vi "MW_AHRS_Paser.vi"(4 "error":errorcluster, 7 "String In":string) -> (0 "error IO":errorcluster, 3 "Output":T1)   [LabVIEW 2015]
panel:
  out "Yaw":dbl
  out "Pitch":dbl
  out "Roll":dbl
  out "Gyro_Z":dbl
  out "Gyro_Y":dbl
  out "Gyro_X":dbl
  out "Acc_X":dbl
  out "Acc_Y":dbl
  out "Acc_Z":dbl
  out "String":string
  # "MW-AHRS 프로그램 이며 센서 출력을 ACC, Gryo, 오일러 출력으로 \n세팅해야 프로그램이 정상적으로 구동 됨"
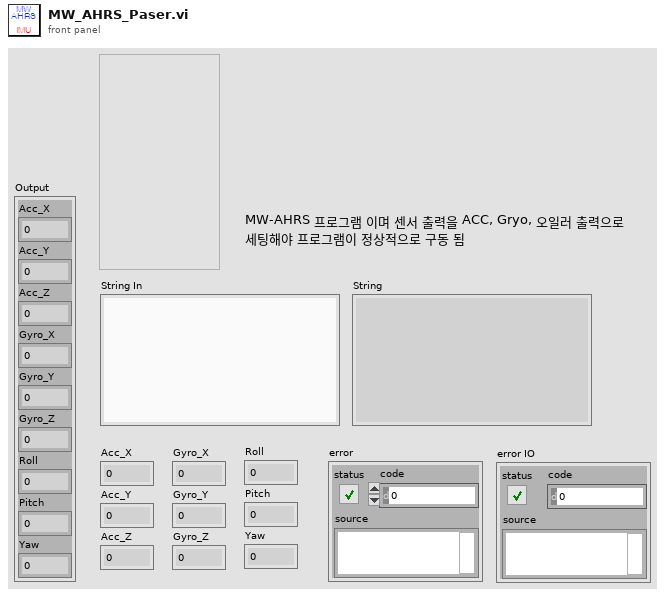
[diagram p1: front panel]
types:
  T1 = cluster{"Acc_X":dbl, "Acc_Y":dbl, "Acc_Z":dbl, "Gyro_X":dbl, "Gyro_Y":dbl, "Gyro_Z":dbl, "Roll":dbl, "Pitch":dbl, "Yaw":dbl}
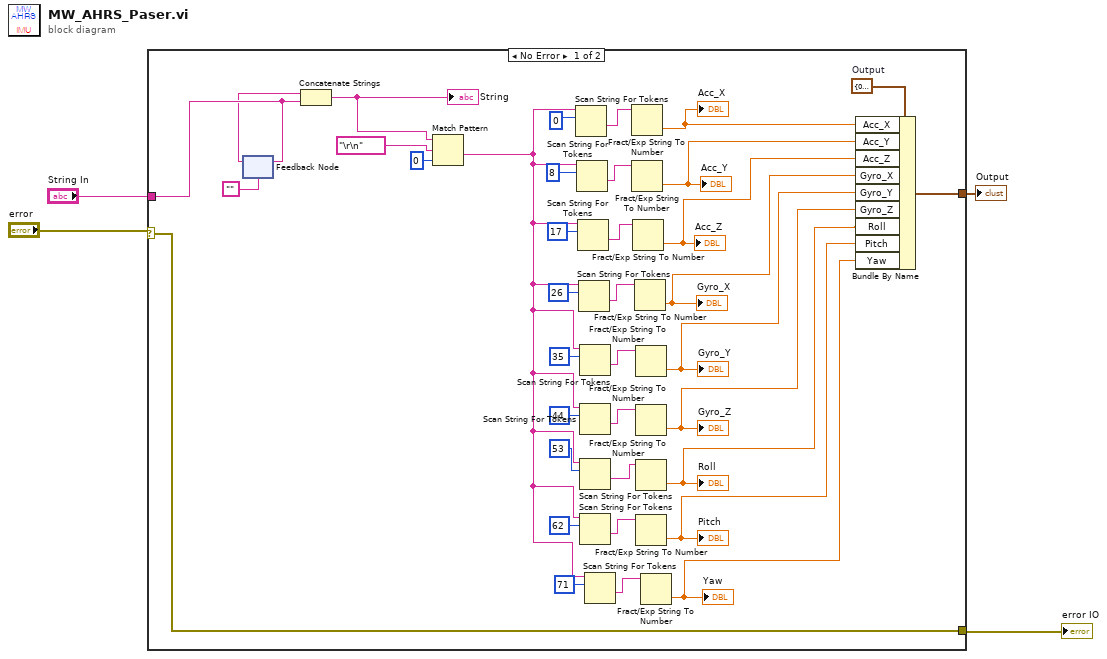
[diagram p0: block diagram]
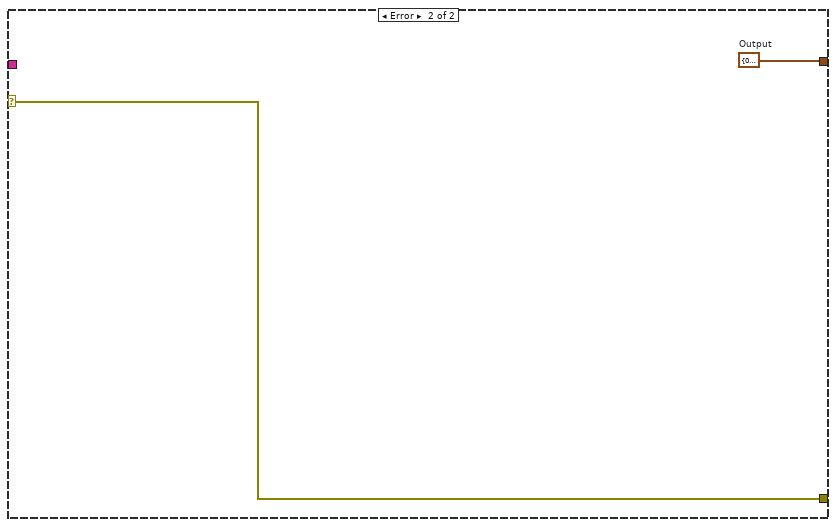
[diagram p2: hidden frame]
diagram:
  n1 = case shown="No Error" "error" {
    selector: "error" -> [w35 w43]
    tunnel: "String In" -> [w41 _]
    tunnel: [w35 w43] -> w2
    tunnel: [w6 w42] -> w1
    frame No Error {
      w16 = T1 {"Acc_X"=0.0, "Acc_Y"=0.0, "Acc_Z"=0.0, "Gyro_X"=0.0, "Gyro_Y"=0.0, "Gyro_Z"=0.0, "Roll"=0.0, "Pitch"=0.0, "Yaw"=0.0}  # Output
      n2 = feedback #1("") -> (w36:string)
      n3 = feedback-in #1(w41) -> ()
      n4 = Concatenate Strings(w36, w41) -> (w38:string)
      "String" <- w38
      n5 = Match Pattern(string=w38, regular expression="\r\n", offset (0)=0) -> (after substring=w5:string)  [unwired: 3 out]
      n6 = Scan String For Tokens(8:0, 9:w5) -> (1:w29:string)  [unwired: 4 in, 3 out]
      n7 = Scan String For Tokens(8:8, 9:w5) -> (1:w30:string)  [unwired: 4 in, 3 out]
      n8 = Scan String For Tokens(8:17, 9:w5) -> (1:w31:string)  [unwired: 4 in, 3 out]
      n9 = Scan String For Tokens(8:26, 9:w5) -> (1:w25:string)  [unwired: 4 in, 3 out]
      n10 = Scan String For Tokens(8:35, 9:w5) -> (1:w26:string)  [unwired: 4 in, 3 out]
      n11 = Scan String For Tokens(8:44, 9:w5) -> (1:w24:string)  [unwired: 4 in, 3 out]
      n12 = Scan String For Tokens(8:53, 9:w5) -> (1:w21:string)  [unwired: 4 in, 3 out]
      n13 = Scan String For Tokens(8:62, 9:w5) -> (1:w19:string)  [unwired: 4 in, 3 out]
      n14 = Scan String For Tokens(8:71, 9:w5) -> (1:w18:string)  [unwired: 4 in, 3 out]
      n15 = Fract/Exp String To Number(string=w29) -> (number=w15:dbl)  [unwired: 3 in, 1 out]
      "Acc_X" <- w15
      n16 = Fract/Exp String To Number(string=w30) -> (number=w14:dbl)  [unwired: 3 in, 1 out]
      "Acc_Y" <- w14
      n17 = Fract/Exp String To Number(string=w31) -> (number=w13:dbl)  [unwired: 3 in, 1 out]
      "Acc_Z" <- w13
      n18 = Fract/Exp String To Number(string=w25) -> (number=w12:dbl)  [unwired: 3 in, 1 out]
      "Gyro_X" <- w12
      n19 = Fract/Exp String To Number(string=w26) -> (number=w11:dbl)  [unwired: 3 in, 1 out]
      "Gyro_Y" <- w11
      n20 = Fract/Exp String To Number(string=w24) -> (number=w10:dbl)  [unwired: 3 in, 1 out]
      "Gyro_Z" <- w10
      n21 = Fract/Exp String To Number(string=w21) -> (number=w9:dbl)  [unwired: 3 in, 1 out]
      "Roll" <- w9
      n22 = Fract/Exp String To Number(string=w19) -> (number=w8:dbl)  [unwired: 3 in, 1 out]
      "Pitch" <- w8
      n23 = Fract/Exp String To Number(string=w18) -> (number=w7:dbl)  [unwired: 3 in, 1 out]
      "Yaw" <- w7
      n24 = Bundle By Name(cluster=w16, "Acc_X"=w15, "Acc_Y"=w14, "Acc_Z"=w13, "Gyro_X"=w12, "Gyro_Y"=w11, "Gyro_Z"=w10, "Roll"=w9, "Pitch"=w8, "Yaw"=w7) -> (w6:T1)
    }
    frame Error {
      w42 = T1 {"Acc_X"=0.0, "Acc_Y"=0.0, "Acc_Z"=0.0, "Gyro_X"=0.0, "Gyro_Y"=0.0, "Gyro_Z"=0.0, "Roll"=0.0, "Pitch"=0.0, "Yaw"=0.0}  # Output
    }
  }
  "error IO" <- w2
  "Output" <- w1
